vi "Display All Channels.vi"(0 "tagged llp packets cluster":T1, 1 "reset":bool, 2 "common resources":T11, 5 "serial channel display parameters":T23[](array[typedef])=[{"virtual channel"=0.0, "payload data type"=enum."Frame Start", "frame skip count"=0, "line skip count"=0, "pixel skip count"=0.0}, {"virtual channel"=0.0, "payload data type"=enum."Frame Start", "frame skip count"=0, "line skip count"=0, "pixel skip count"=0.0}, {"virtual channel"=0.0, "payload data type"=enum."Frame Start", "frame skip count"=0, "line skip count"=0, "pixel skip count"=0.0}, {"virtual channel"=0.0, "payload data type"=enum."Frame Start", "frame skip count"=0, "line skip count"=0, "pixel skip count"=0.0}, {"virtual channel"=0.0, "payload data type"=enum."Frame Start", "frame skip count"=0, "line skip count"=0, "pixel skip count"=0.0}, {"virtual channel"=0.0, "payload data type"=enum."Frame Start", "frame skip count"=0, "line skip count"=0, "pixel skip count"=0.0}, {"virtual channel"=0.0, "payload data type"=enum."Frame Start", "frame skip count"=0, "line skip count"=0, "pixel skip count"=0.0}, {"virtual channel"=0.0, "payload data type"=enum."Frame Start", "frame skip count"=0, "line skip count"=0, "pixel skip count"=0.0}], 7 "display serial channel selectors":fxp<+,3,3>[](array[numeric])=[0.0, 0.0, 0.0, 0.0, 0.0, 0.0, 0.0, 0.0], 9 "input valid":bool[](array[boolean])=[FALSE, FALSE, FALSE, FALSE, FALSE, FALSE, FALSE, FALSE], 11 "enabled display channels":bool[](array[boolean])=[FALSE, FALSE, FALSE, FALSE, FALSE, FALSE, FALSE, FALSE], 12 "gate display until frame complete":bool, 13 "num available display channels":fxp<+,4,4>=2.0) -> (4 "display channel status":T22[](array[typedef]), 14 "ready for input":bool[](array[boolean]))   [LabVIEW 2020, in "GettingStarted_Common_148X_FPGA.lvlib"]
uses:
  GettingStarted_Common_148X_FPGA.lvlib
  <instrlib>/FlexRIO/CSI-2/v2/FPGA/Types/Display Parameters.ctl
  <instrlib>/FlexRIO/CSI-2/v2/Common/Types/LLP Data Type.ctl
  Types/Display Channel Status.ctl
  Types/Common Resources.ctl
  <instrlib>/_niInstr/Memory/v1/FPGA/DRAM/niInstr Memory DRAM v1 FPGA.lvclass
  <instrlib>/FlexRIO/CSI-2/v2/FPGA/Types/Sync Pulse Resources.ctl
  Types/Serial Channel Resources.ctl
  Types/Single Serial Channel Resources.ctl
  <instrlib>/FlexRIO/CSI-2/v2/FPGA/DRAM Manager/Private/DRAM Manager.ctl
  <instrlib>/FlexRIO/CSI-2/v2/FPGA/DRAM Manager/Private/Common/DRAM Manager Registers.ctl
  <instrlib>/FlexRIO/CSI-2/v2/FPGA/DRAM Manager/Private/Common/Handshake Registers.ctl
  <instrlib>/FlexRIO/CSI-2/v2/FPGA/DRAM Manager/Private/Common/DRAM Manager FIFOs.ctl
  <instrlib>/FlexRIO/CSI-2/v2/FPGA/DRAM Manager/Private/Common/Write Data FIFO Ref.ctl
  <instrlib>/FlexRIO/CSI-2/v2/FPGA/DRAM Manager/Private/Common/Read Request Metadata FIFO Ref.ctl
  <instrlib>/FlexRIO/CSI-2/v2/FPGA/DRAM Manager/Private/Common/Read Data FIFO Ref.ctl
  Types/Tagged LLP Packets Cluster.ctl
  <instrlib>/FlexRIO/CSI-2/v2/FPGA/Types/Tagged LLP Packet.ctl
  <instrlib>/FlexRIO/CSI-2/v2/FPGA/Types/FPGA LLP Packet Tag.ctl
  <instrlib>/FlexRIO/CSI-2/v2/FPGA/Types/FPGA LLP Packet Timestamp.ctl
  <instrlib>/FlexRIO/CSI-2/v2/FPGA/Types/Timestamp ID.ctl
  <instrlib>/FlexRIO/CSI-2/v2/FPGA/Types/FPGA LLP Packet Size.ctl
  <instrlib>/FlexRIO/CSI-2/v2/FPGA/Types/LLP Packet.ctl
  <instrlib>/FlexRIO/CSI-2/v2/FPGA/Types/LLP Packet Header.ctl
  <instrlib>/FlexRIO/CSI-2/v2/FPGA/Types/LLP Packet Payload.ctl
  <instrlib>/FlexRIO/CSI-2/v2/FPGA/Types/LLP Packet Footer.ctl
  Types/Display Channel Resources.ctl
  <instrlib>/_niInstr/Basic Elements/v1/FPGA/niInstr Basic Elements v1 FPGA.lvlib
  <instrlib>/FlexRIO/CSI-2/v2/Common/NI CSI-2 API Common v2.lvlib
  <instrlib>/FlexRIO/CSI-2/v2/FPGA/NI CSI-2 API FPGA v2.lvlib
  <instrlib>/FlexRIO/CSI-2/v2/FPGA/DRAM Manager/DRAM Manager v2.lvlib
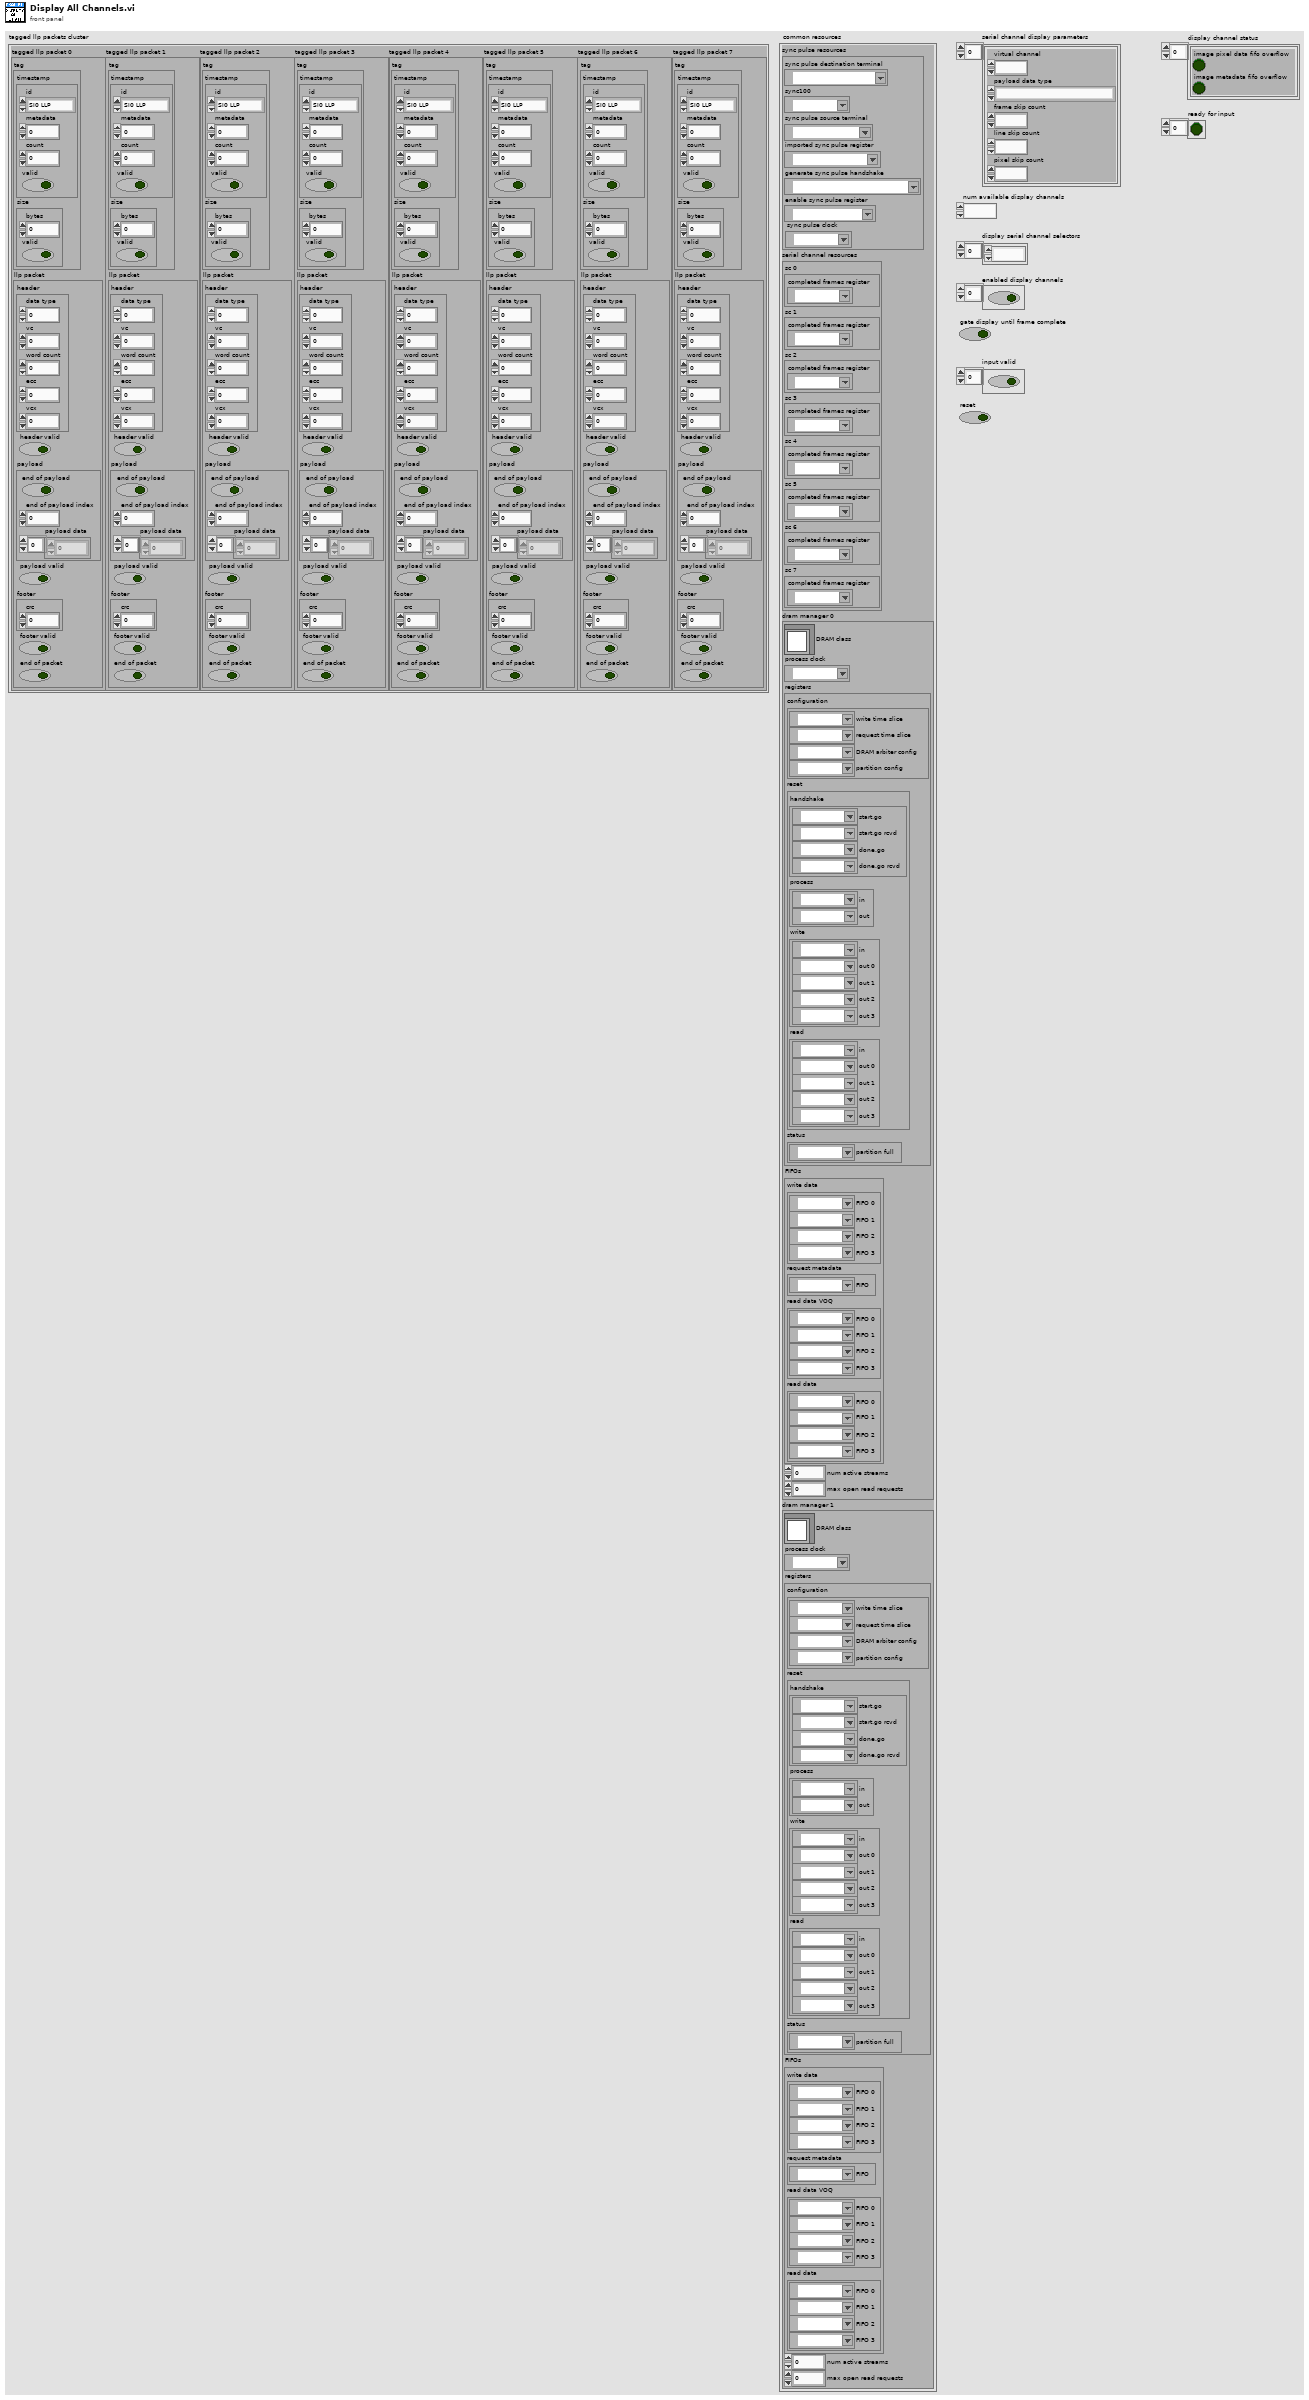
[diagram p1: front panel]
types:
  T1 = typedef "GettingStarted_Common_148X_FPGA.lvlib/Tagged LLP Packets Cluster.ctl" = cluster{"tagged llp packet 0":T2, "tagged llp packet 1":T2, "tagged llp packet 2":T2, "tagged llp packet 3":T2, "tagged llp packet 4":T2, "tagged llp packet 5":T2, "tagged llp packet 6":T2, "tagged llp packet 7":T2}
  T2 = typedef "NI CSI-2 API FPGA v2.lvlib/Tagged LLP Packet.ctl" = cluster{"tag":T3, "llp packet":T7}
  T3 = typedef "NI CSI-2 API FPGA v2.lvlib/FPGA LLP Packet Tag.ctl" = cluster{"timestamp":T4, "size":T6}
  T4 = typedef "NI CSI-2 API FPGA v2.lvlib/FPGA LLP Packet Timestamp.ctl" = cluster{"valid":bool, "count":fxp<+,50,50>, "id":T5, "metadata":u8}
  T5 = typedef "NI CSI-2 API FPGA v2.lvlib/Timestamp ID.ctl" = enum8{"SI0 LLP", "SI1 LLP", "SI2 LLP", "SI3 LLP", "SI4 LLP", "SI5 LLP", "SI6 LLP", "SI7 LLP", "SO0 LLP", "SO1 LLP", "SO2 LLP", "SO3 LLP", "SO4 LLP", "SO5 LLP", "SO6 LLP", "SO7 LLP", "Ser0 GPIO Bank", "Ser1 GPIO Bank", "Ser2 GPIO Bank", "Ser3 GPIO Bank", "Ser4 GPIO Bank", "Ser5 GPIO Bank", "Ser6 GPIO Bank", "Ser7 GPIO Bank", "Des0 GPIO Bank", "Des1 GPIO Bank", "Des2 GPIO Bank", "Des3 GPIO Bank", "Des4 GPIO Bank", "Des5 GPIO Bank", "Des6 GPIO Bank", "Des7 GPIO Bank", "User0", "User1", "User2", "User3", "User4", "User5", "User6", "User7", "User8", "User9", "User10", "User11", "User12", "User13", "User14", "User15", "User16", "User17", "User18", "User19", "User20", "User21", "User22", "User23", "User24", "User25", "User26", "User27", "User28", "User29", "User30", "User31"}
  T6 = typedef "NI CSI-2 API FPGA v2.lvlib/FPGA LLP Packet Size.ctl" = cluster{"bytes":fxp<+,17,17>, "valid":bool}
  T7 = typedef "NI CSI-2 API FPGA v2.lvlib/LLP Packet.ctl" = cluster{"header":T8, "header valid":bool, "payload":T9, "payload valid":bool, "footer":T10, "footer valid":bool, "end of packet":bool}
  T8 = typedef "NI CSI-2 API FPGA v2.lvlib/LLP Packet Header.ctl" = cluster{"word count":u16, "ecc":fxp<+,6,6>, "vcx":fxp<+,2,2>, "data type":fxp<+,6,6>, "vc":fxp<+,2,2>}
  T9 = typedef "NI CSI-2 API FPGA v2.lvlib/LLP Packet Payload.ctl" = cluster{"end of payload":bool, "end of payload index":fxp<+,3,3>, "payload data":u8[]}
  T10 = typedef "NI CSI-2 API FPGA v2.lvlib/LLP Packet Footer.ctl" = cluster{"crc":u16}
  T11 = typedef "GettingStarted_Common_148X_FPGA.lvlib/Common Resources.ctl" = cluster{"sync pulse resources":T12, "serial channel resources":T13, "dram manager 0":T15, "dram manager 1":T15}
  T12 = typedef "NI CSI-2 API FPGA v2.lvlib/Sync Pulse Resources.ctl" = cluster{"sync pulse destination terminal":refnum<k21>, "sync100":refnum<k21>, "sync pulse source terminal":refnum<k21>, "imported sync pulse register":refnum<k21>, "generate sync pulse handshake":refnum<k21>, "enable sync pulse register":refnum<k21>, "sync pulse clock":refnum<k21>}
  T13 = typedef "GettingStarted_Common_148X_FPGA.lvlib/Serial Channel Resources.ctl" = cluster{"sc 0":T14, "sc 1":T14, "sc 2":T14, "sc 3":T14, "sc 4":T14, "sc 5":T14, "sc 6":T14, "sc 7":T14}
  T14 = typedef "GettingStarted_Common_148X_FPGA.lvlib/Single Serial Channel Resources.ctl" = cluster{"completed frames register":refnum<k21>}
  T15 = typedef "DRAM Manager v2.lvlib/DRAM Manager.ctl" = cluster{"DRAM class":refnum<class "niInstr Memory DRAM v1 FPGA.lvclass">, "process clock":refnum<k21>, "registers":T16, "FIFOs":T18, "num active streams":fxp<+,3,3>, "max open read requests":u16}
  T16 = typedef "DRAM Manager v2.lvlib/DRAM Manager Registers.ctl" = cluster{"configuration":cluster{"write time slice":refnum<k21>, "request time slice":refnum<k21>, "DRAM arbiter config":refnum<k21>, "partition config":refnum<k21>}, "reset":cluster{"handshake":T17, "process":cluster{"in":refnum<k21>, "out":refnum<k21>}, "write":cluster{"in":refnum<k21>, "out 0":refnum<k21>, "out 1":refnum<k21>, "out 2":refnum<k21>, "out 3":refnum<k21>}, "read":cluster{"in":refnum<k21>, "out 0":refnum<k21>, "out 1":refnum<k21>, "out 2":refnum<k21>, "out 3":refnum<k21>}}, "status":cluster{"partition full":refnum<k21>}}
  T17 = typedef "DRAM Manager v2.lvlib/Handshake Registers.ctl" = cluster{"start.go":refnum<k21>, "start.go rcvd":refnum<k21>, "done.go":refnum<k21>, "done.go rcvd":refnum<k21>}
  T18 = typedef "DRAM Manager v2.lvlib/DRAM Manager FIFOs.ctl" = cluster{"write data":cluster{"FIFO 0":T19, "FIFO 1":T19, "FIFO 2":T19, "FIFO 3":T19}, "request metadata":cluster{"FIFO":T20}, "read data VOQ":cluster{"FIFO 0":T21, "FIFO 1":T21, "FIFO 2":T21, "FIFO 3":T21}, "read data":cluster{"FIFO 0":T21, "FIFO 1":T21, "FIFO 2":T21, "FIFO 3":T21}}
  T19 = typedef "DRAM Manager v2.lvlib/Write Data FIFO Ref.ctl" = refnum<k21>
  T20 = typedef "DRAM Manager v2.lvlib/Read Request Metadata FIFO Ref.ctl" = refnum<k21>
  T21 = typedef "DRAM Manager v2.lvlib/Read Data FIFO Ref.ctl" = refnum<k21>
  T22 = typedef "GettingStarted_Common_148X_FPGA.lvlib/Display Channel Status.ctl" = cluster{"image pixel data fifo overflow":bool, "image metadata fifo overflow":bool}
  T23 = typedef "NI CSI-2 API FPGA v2.lvlib/Display Parameters.ctl" = cluster{"virtual channel":fxp<+,4,4>, "payload data type":T24, "frame skip count":u16, "line skip count":u8, "pixel skip count":fxp<+,5,5>}
  T24 = typedef "NI CSI-2 API Common v2.lvlib/LLP Data Type.ctl" = enum8{"Frame Start", "Frame End", "Line Start", "Line End", "End of Transmission", "Reserved 0", "Reserved 1", "Reserved 2", "Generic Short Packet 1", "Generic Short Packet 2", "Generic Short Packet 3", "Generic Short Packet 4", "Generic Short Packet 5", "Generic Short Packet 6", "Generic Short Packet 7", "Generic Short Packet 8", "Null", "Blanking Data", "Embedded 8-bit non Image Data", "Generic Long Packet 1", "Generic Long Packet 2", "Generic Long Packet 3", "Generic Long Packet 4", "Reserved 3", "YUV420 8-bit", "YUV420 10-bit", "Legacy YUV420 8-bit", "Reserved 4", "YUV420 8-bit Chroma Shifted", "YUV420 10-bit Chroma Shifted", "YUV422 8-bit", "YUV422 10-bit", "RGB444", "RGB555", "RGB565", "RGB666", "RGB888", "Reserved 5", "Reserved 6", "RAW 24", "RAW 6", "RAW 7", "RAW 8", "RAW 10", "RAW 12", "RAW 14", "RAW 16", "RAW 20", "User Defined 8-bit Data 1", "User Defined 8-bit Data 2", "User Defined 8-bit Data 3", "User Defined 8-bit Data 4", "User Defined 8-bit Data 5", "User Defined 8-bit Data 6", "User Defined 8-bit Data 7", "User Defined 8-bit Data 8", "USL Command", "Reserved 7", "Reserved 8", "Reserved 9", "Reserved 10", "Reserved 11", "Reserved 12", "LRTE EPD Spacer"}
  T25 = typedef "GettingStarted_Common_148X_FPGA.lvlib/Display Channel Resources.ctl" = cluster{"image pixel data dma fifo x8":refnum<k21>, "image pixel data dma fifo x16":refnum<k21>, "image metadata dma fifo":refnum<k21>, "serial channel resources":T13}
  T26 = cluster{"gate display until frame complete":bool, "reset":bool, "serial channel display parameters":T23[], "tagged llp packets cluster":T1, "output valid":bool[], "display channel resources":cluster{"display resources 0":T25, "display resources 1":T25, "display resources 2":T25, "display resources 3":T25, "display resources 4":T25, "display resources 5":T25, "display resources 6":T25, "display resources 7":T25}}
  T27 = cluster{"channel selector":fxp<+,3,3>, "enabled display channels":bool}
  T28 = cluster{"display resources 0":T25, "display resources 1":T25, "display resources 2":T25, "display resources 3":T25, "display resources 4":T25, "display resources 5":T25, "display resources 6":T25, "display resources 7":T25}
  T29 = cluster{"display channel status":T22, "selected channel":fxp<+,3,3>, "ready for input":bool, "enabled display channels":bool}
  T30 = cluster{"display channel status":T22, "selected channel":fxp<+,3,3>, "ready for input":bool, "enabled display channels":bool}[]
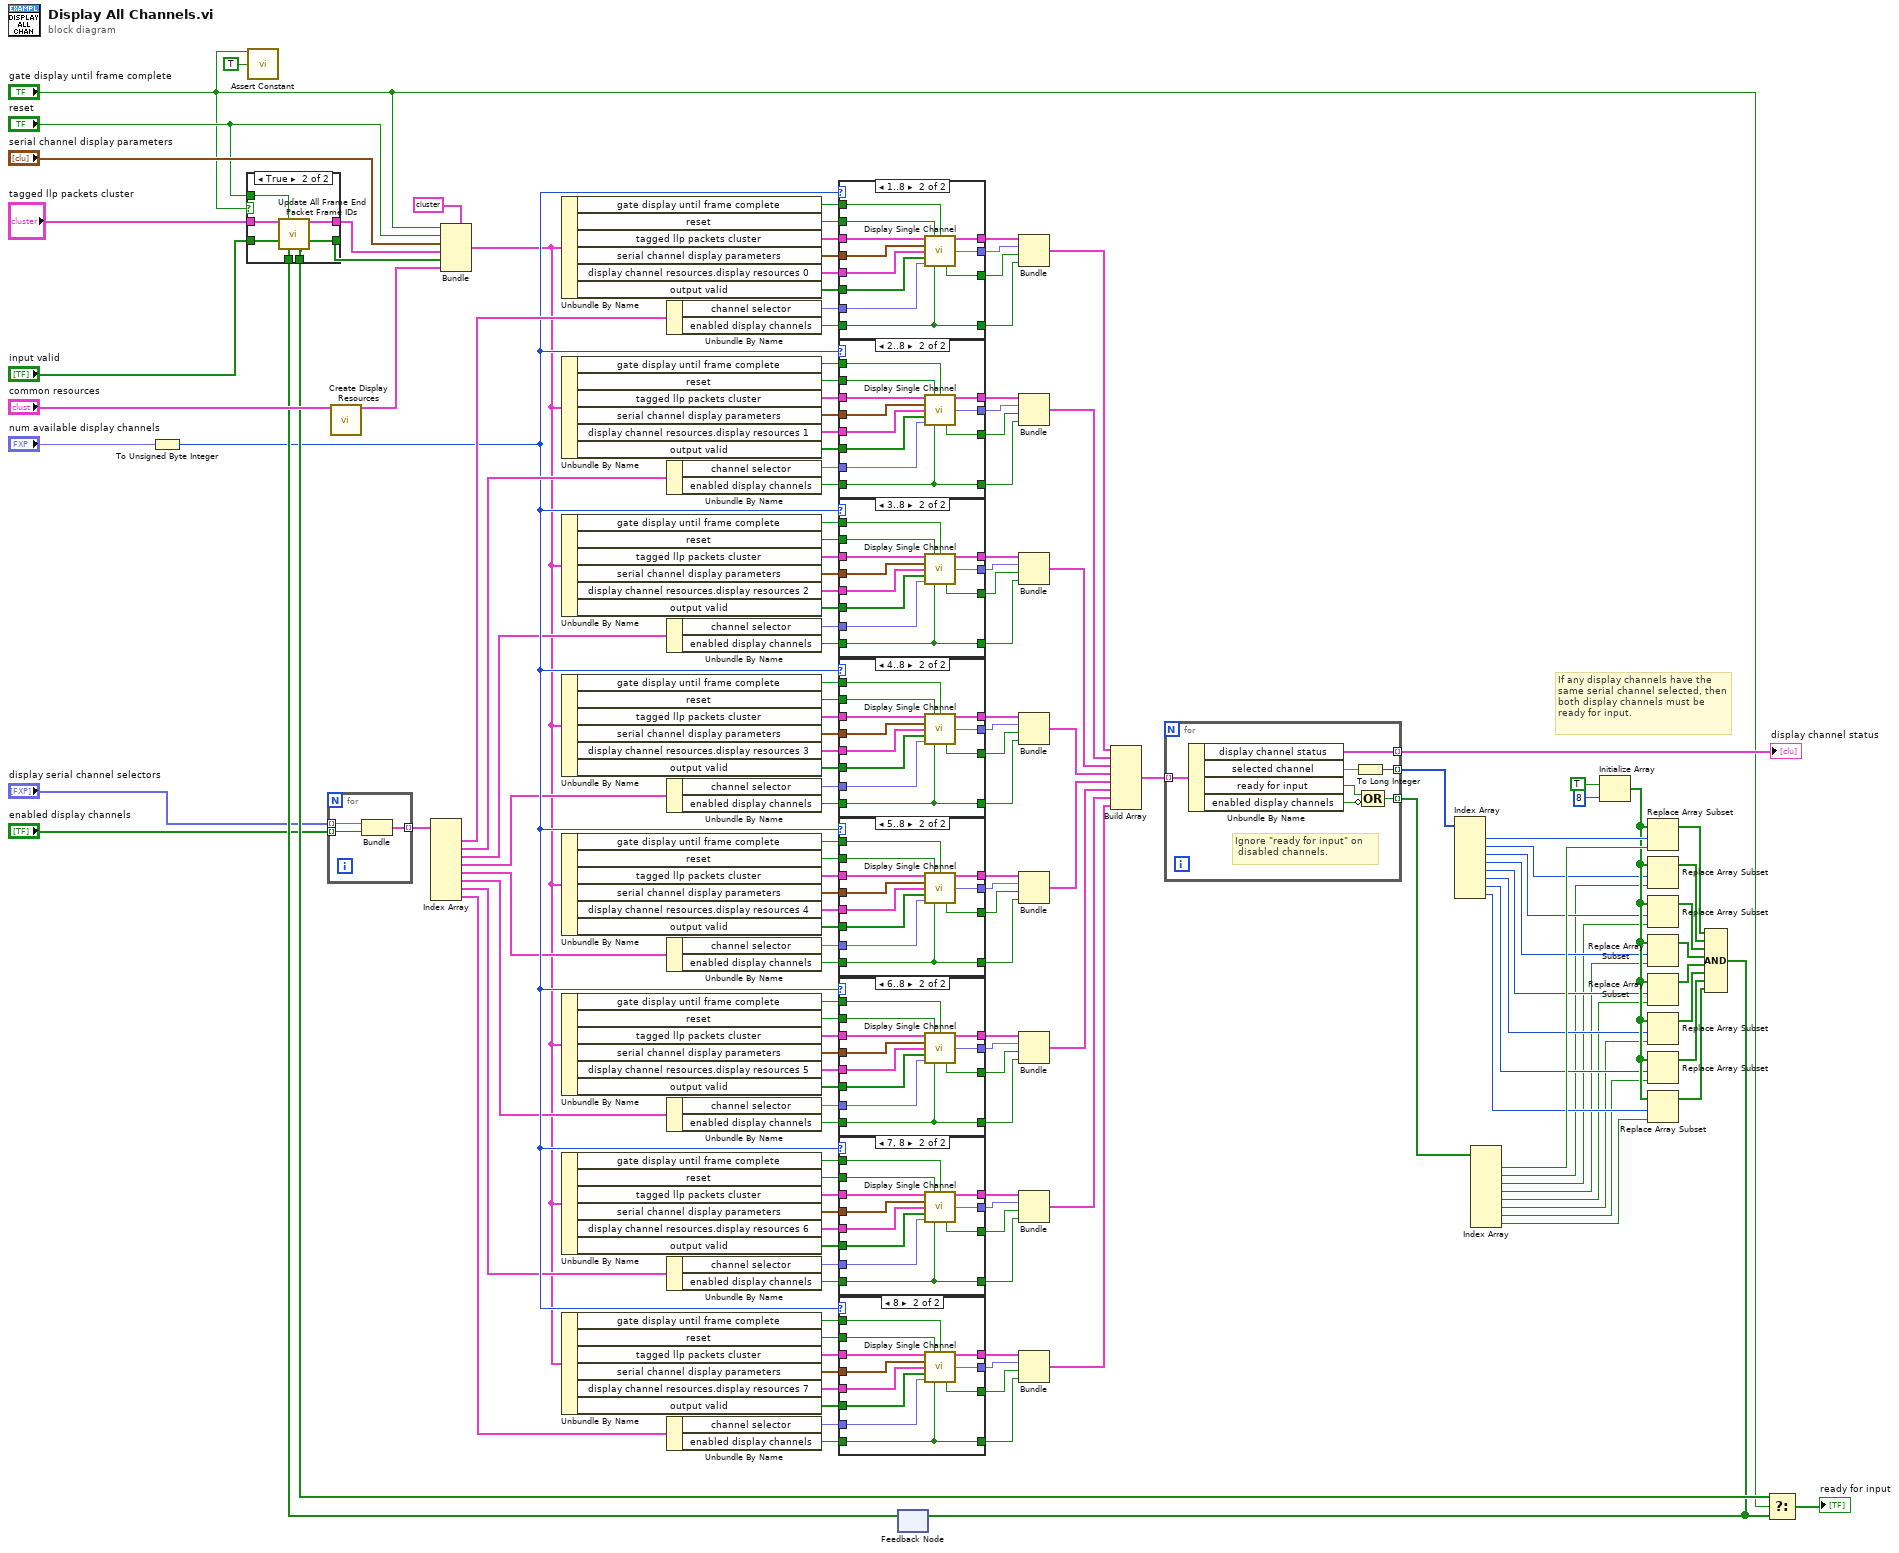
[diagram p0: block diagram]
diagram:
  # "If any display channels have the same serial channel selected, then both display channels must be ready for input."
  n1 = To Unsigned Byte Integer(number="num available display channels") -> (unsigned 8bit integer=w85:u8)
  n2 = call <instrlib>:"Assert Constant.vi"("constant terminal"="gate display until frame complete", "enable show error"=TRUE) -> ()  [unwired: 14 in]
  n3 = for {
    tunnel: "enabled display channels" -> [w166] mode=indexing
    tunnel: "display serial channel selectors" -> [w167] mode=indexing
    tunnel: [w165] -> w105 mode=indexing
    n4 = Bundle("channel selector"=w167, "enabled display channels"=w166) -> (w165:T27)  [unwired: 1 in]
  }
  n5 = call "Create Display Resources.vi"("common resources"="common resources") -> ("display channel resources"=w112:T28)  [unwired: 14 in]
  n6 = Index Array(array=w105) -> (element #1=w104:T27, element #2=w86:T27, element #3=w18:T27, element #4=w17:T27, element #5=w16:T27, element #6=w13:T27, element #7=w15:T27, element #8=w14:T27)  [unwired: 8 in]
  n7 = Unbundle By Name(w104) -> ("channel selector"=w102:fxp<+,3,3>, "enabled display channels"=w103:bool)
  n8 = Unbundle By Name(w86) -> ("channel selector"=w91:fxp<+,3,3>, "enabled display channels"=w90:bool)
  n9 = Unbundle By Name(w18) -> ("channel selector"=w73:fxp<+,3,3>, "enabled display channels"=w72:bool)
  n10 = Unbundle By Name(w17) -> ("channel selector"=w66:fxp<+,3,3>, "enabled display channels"=w65:bool)
  n11 = Unbundle By Name(w16) -> ("channel selector"=w50:fxp<+,3,3>, "enabled display channels"=w49:bool)
  n12 = Unbundle By Name(w13) -> ("channel selector"=w43:fxp<+,3,3>, "enabled display channels"=w42:bool)
  n13 = Unbundle By Name(w15) -> ("channel selector"=w27:fxp<+,3,3>, "enabled display channels"=w26:bool)
  n14 = Unbundle By Name(w14) -> ("channel selector"=w20:fxp<+,3,3>, "enabled display channels"=w19:bool)
  n15 = feedback #1() -> (w159:bool[])  [unwired: 1 in]
  n16 = case shown="True" "gate display until frame complete" {
    tunnel: "reset" -> [_ w176]
    tunnel: "input valid" -> [w168 w175]
    tunnel: [w168 w174] -> w113
    tunnel: "tagged llp packets cluster" -> [w169 w173]
    tunnel: [w169 w172] -> w110
    tunnel: [_ w171] -> w158
    tunnel: w159 -> [_ w170]
    frame False {
    }
    frame True {
      n17 = call "Update All Frame End Packet Frame IDs.vi"("tagged llp packets cluster"=w173, "reset"=w176, "input valid"=w175, "ready for output"=w170) -> ("tagged llp packets cluster"=w172:T1, "output valid"=w174:bool[], "ready for input"=w171:bool[])  [unwired: 9 in]
    }
  }
  n18 = Bundle(cluster=T26 {"gate display until frame complete"=FALSE, "reset"=FALSE, "serial channel display parameters"=[{"virtual channel"=0.0, "payload data type"=enum."Frame Start", "frame skip count"=0, "line skip count"=0, "pixel skip count"=0.0}, {"virtual channel"=0.0, "payload data type"=enum."Frame Start", "frame skip count"=0, "line skip count"=0, "pixel skip count"=0.0}, {"virtual channel"=0.0, "payload data type"=enum."Frame Start", "frame skip count"=0, "line skip count"=0, "pixel skip count"=0.0}, {"virtual channel"=0.0, "payload data type"=enum."Frame Start", "frame skip count"=0, "line skip count"=0, "pixel skip count"=0.0}, {"virtual channel"=0.0, "payload data type"=enum."Frame Start", "frame skip count"=0, "line skip count"=0, "pixel skip count"=0.0}, {"virtual channel"=0.0, "payload data type"=enum."Frame Start", "frame skip count"=0, "line skip count"=0, "pixel skip count"=0.0}, {"virtual channel"=0.0, "payload data type"=enum."Frame Start", "frame skip count"=0, "line skip count"=0, "pixel skip count"=0.0}, {"virtual channel"=0.0, "payload data type"=enum."Frame Start", "frame skip count"=0, "line skip count"=0, "pixel skip count"=0.0}], "tagged llp packets cluster"={"tagged llp packet 0"={"tag"={"timestamp"={"valid"=FALSE, "count"=0.0, "id"=enum."SI0 LLP", "metadata"=0}, "size"={"bytes"=0.0, "valid"=FALSE}}, "llp packet"={"header"={"word count"=0, "ecc"=0.0, "vcx"=0.0, "data type"=0.0, "vc"=0.0}, "header valid"=FALSE, "payload"={"end of payload"=FALSE, "end of payload index"=0.0, "payload data"=[]}, "payload valid"=FALSE, "footer"={"crc"=0}, "footer valid"=FALSE, "end of packet"=FALSE}}, "tagged llp packet 1"={"tag"={"timestamp"={"valid"=FALSE, "count"=0.0, "id"=enum."SI0 LLP", "metadata"=0}, "size"={"bytes"=0.0, "valid"=FALSE}}, "llp packet"={"header"={"word count"=0, "ecc"=0.0, "vcx"=0.0, "data type"=0.0, "vc"=0.0}, "header valid"=FALSE, "payload"={"end of payload"=FALSE, "end of payload index"=0.0, "payload data"=[]}, "payload valid"=FALSE, "footer"={"crc"=0}, "footer valid"=FALSE, "end of packet"=FALSE}}, "tagged llp packet 2"={"tag"={"timestamp"={"valid"=FALSE, "count"=0.0, "id"=enum."SI0 LLP", "metadata"=0}, "size"={"bytes"=0.0, "valid"=FALSE}}, "llp packet"={"header"={"word count"=0, "ecc"=0.0, "vcx"=0.0, "data type"=0.0, "vc"=0.0}, "header valid"=FALSE, "payload"={"end of payload"=FALSE, "end of payload index"=0.0, "payload data"=[]}, "payload valid"=FALSE, "footer"={"crc"=0}, "footer valid"=FALSE, "end of packet"=FALSE}}, "tagged llp packet 3"={"tag"={"timestamp"={"valid"=FALSE, "count"=0.0, "id"=enum."SI0 LLP", "metadata"=0}, "size"={"bytes"=0.0, "valid"=FALSE}}, "llp packet"={"header"={"word count"=0, "ecc"=0.0, "vcx"=0.0, "data type"=0.0, "vc"=0.0}, "header valid"=FALSE, "payload"={"end of payload"=FALSE, "end of payload index"=0.0, "payload data"=[]}, "payload valid"=FALSE, "footer"={"crc"=0}, "footer valid"=FALSE, "end of packet"=FALSE}}, "tagged llp packet 4"={"tag"={"timestamp"={"valid"=FALSE, "count"=0.0, "id"=enum."SI0 LLP", "metadata"=0}, "size"={"bytes"=0.0, "valid"=FALSE}}, "llp packet"={"header"={"word count"=0, "ecc"=0.0, "vcx"=0.0, "data type"=0.0, "vc"=0.0}, "header valid"=FALSE, "payload"={"end of payload"=FALSE, "end of payload index"=0.0, "payload data"=[]}, "payload valid"=FALSE, "footer"={"crc"=0}, "footer valid"=FALSE, "end of packet"=FALSE}}, "tagged llp packet 5"={"tag"={"timestamp"={"valid"=FALSE, "count"=0.0, "id"=enum."SI0 LLP", "metadata"=0}, "size"={"bytes"=0.0, "valid"=FALSE}}, "llp packet"={"header"={"word count"=0, "ecc"=0.0, "vcx"=0.0, "data type"=0.0, "vc"=0.0}, "header valid"=FALSE, "payload"={"end of payload"=FALSE, "end of payload index"=0.0, "payload data"=[]}, "payload valid"=FALSE, "footer"={"crc"=0}, "footer valid"=FALSE, "end of packet"=FALSE}}, "tagged llp packet 6"={"tag"={"timestamp"={"valid"=FALSE, "count"=0.0, "id"=enum."SI0 LLP", "metadata"=0}, "size"={"bytes"=0.0, "valid"=FALSE}}, "llp packet"={"header"={"word count"=0, "ecc"=0.0, "vcx"=0.0, "data type"=0.0, "vc"=0.0}, "header valid"=FALSE, "payload"={"end of payload"=FALSE, "end of payload index"=0.0, "payload data"=[]}, "payload valid"=FALSE, "footer"={"crc"=0}, "footer valid"=FALSE, "end of packet"=FALSE}}, "tagged llp packet 7"={"tag"={"timestamp"={"valid"=FALSE, "count"=0.0, "id"=enum."SI0 LLP", "metadata"=0}, "size"={"bytes"=0.0, "valid"=FALSE}}, "llp packet"={"header"={"word count"=0, "ecc"=0.0, "vcx"=0.0, "data type"=0.0, "vc"=0.0}, "header valid"=FALSE, "payload"={"end of payload"=FALSE, "end of payload index"=0.0, "payload data"=[]}, "payload valid"=FALSE, "footer"={"crc"=0}, "footer valid"=FALSE, "end of packet"=FALSE}}}, "output valid"=[FALSE, FALSE, FALSE, FALSE, FALSE, FALSE, FALSE, FALSE], "display channel resources"={"display resources 0"={"image pixel data dma fifo x8"="", "image pixel data dma fifo x16"="", "image metadata dma fifo"="", "serial channel resources"={"sc 0"={"completed frames register"=""}, "sc 1"={"completed frames register"=""}, "sc 2"={"completed frames register"=""}, "sc 3"={"completed frames register"=""}, "sc 4"={"completed frames register"=""}, "sc 5"={"completed frames register"=""}, "sc 6"={"completed frames register"=""}, "sc 7"={"completed frames register"=""}}}, "display resources 1"={"image pixel data dma fifo x8"="", "image pixel data dma fifo x16"="", "image metadata dma fifo"="", "serial channel resources"={"sc 0"={"completed frames register"=""}, "sc 1"={"completed frames register"=""}, "sc 2"={"completed frames register"=""}, "sc 3"={"completed frames register"=""}, "sc 4"={"completed frames register"=""}, "sc 5"={"completed frames register"=""}, "sc 6"={"completed frames register"=""}, "sc 7"={"completed frames register"=""}}}, "display resources 2"={"image pixel data dma fifo x8"="", "image pixel data dma fifo x16"="", "image metadata dma fifo"="", "serial channel resources"={"sc 0"={"completed frames register"=""}, "sc 1"={"completed frames register"=""}, "sc 2"={"completed frames register"=""}, "sc 3"={"completed frames register"=""}, "sc 4"={"completed frames register"=""}, "sc 5"={"completed frames register"=""}, "sc 6"={"completed frames register"=""}, "sc 7"={"completed frames register"=""}}}, "display resources 3"={"image pixel data dma fifo x8"="", "image pixel data dma fifo x16"="", "image metadata dma fifo"="", "serial channel resources"={"sc 0"={"completed frames register"=""}, "sc 1"={"completed frames register"=""}, "sc 2"={"completed frames register"=""}, "sc 3"={"completed frames register"=""}, "sc 4"={"completed frames register"=""}, "sc 5"={"completed frames register"=""}, "sc 6"={"completed frames register"=""}, "sc 7"={"completed frames register"=""}}}, "display resources 4"={"image pixel data dma fifo x8"="", "image pixel data dma fifo x16"="", "image metadata dma fifo"="", "serial channel resources"={"sc 0"={"completed frames register"=""}, "sc 1"={"completed frames register"=""}, "sc 2"={"completed frames register"=""}, "sc 3"={"completed frames register"=""}, "sc 4"={"completed frames register"=""}, "sc 5"={"completed frames register"=""}, "sc 6"={"completed frames register"=""}, "sc 7"={"completed frames register"=""}}}, "display resources 5"={"image pixel data dma fifo x8"="", "image pixel data dma fifo x16"="", "image metadata dma fifo"="", "serial channel resources"={"sc 0"={"completed frames register"=""}, "sc 1"={"completed frames register"=""}, "sc 2"={"completed frames register"=""}, "sc 3"={"completed frames register"=""}, "sc 4"={"completed frames register"=""}, "sc 5"={"completed frames register"=""}, "sc 6"={"completed frames register"=""}, "sc 7"={"completed frames register"=""}}}, "display resources 6"={"image pixel data dma fifo x8"="", "image pixel data dma fifo x16"="", "image metadata dma fifo"="", "serial channel resources"={"sc 0"={"completed frames register"=""}, "sc 1"={"completed frames register"=""}, "sc 2"={"completed frames register"=""}, "sc 3"={"completed frames register"=""}, "sc 4"={"completed frames register"=""}, "sc 5"={"completed frames register"=""}, "sc 6"={"completed frames register"=""}, "sc 7"={"completed frames register"=""}}}, "display resources 7"={"image pixel data dma fifo x8"="", "image pixel data dma fifo x16"="", "image metadata dma fifo"="", "serial channel resources"={"sc 0"={"completed frames register"=""}, "sc 1"={"completed frames register"=""}, "sc 2"={"completed frames register"=""}, "sc 3"={"completed frames register"=""}, "sc 4"={"completed frames register"=""}, "sc 5"={"completed frames register"=""}, "sc 6"={"completed frames register"=""}, "sc 7"={"completed frames register"=""}}}}} ("output cluster"), "gate display until frame complete"="gate display until frame complete", "reset"="reset", "serial channel display parameters"="serial channel display parameters", "tagged llp packets cluster"=w110, "output valid"=w113, "display channel resources"=w112) -> (w12:T26)
  n19 = Unbundle By Name(w12) -> ("gate display until frame complete"=w99:bool, "reset"=w98:bool, "tagged llp packets cluster"=w109:T1, "serial channel display parameters"=w108:T23[], "display channel resources.display resources 0"=w107:T25, "output valid"=w106:bool[])
  n20 = Unbundle By Name(w12) -> ("gate display until frame complete"=w97:bool, "reset"=w96:bool, "tagged llp packets cluster"=w95:T1, "serial channel display parameters"=w94:T23[], "display channel resources.display resources 1"=w93:T25, "output valid"=w92:bool[])
  n21 = Unbundle By Name(w12) -> ("gate display until frame complete"=w84:bool, "reset"=w78:bool, "tagged llp packets cluster"=w77:T1, "serial channel display parameters"=w76:T23[], "display channel resources.display resources 2"=w75:T25, "output valid"=w74:bool[])
  n22 = Unbundle By Name(w12) -> ("gate display until frame complete"=w83:bool, "reset"=w71:bool, "tagged llp packets cluster"=w70:T1, "serial channel display parameters"=w69:T23[], "display channel resources.display resources 3"=w68:T25, "output valid"=w67:bool[])
  n23 = Unbundle By Name(w12) -> ("gate display until frame complete"=w82:bool, "reset"=w55:bool, "tagged llp packets cluster"=w54:T1, "serial channel display parameters"=w53:T23[], "display channel resources.display resources 4"=w52:T25, "output valid"=w51:bool[])
  n24 = Unbundle By Name(w12) -> ("gate display until frame complete"=w81:bool, "reset"=w48:bool, "tagged llp packets cluster"=w47:T1, "serial channel display parameters"=w46:T23[], "display channel resources.display resources 5"=w45:T25, "output valid"=w44:bool[])
  n25 = Unbundle By Name(w12) -> ("gate display until frame complete"=w79:bool, "reset"=w32:bool, "tagged llp packets cluster"=w31:T1, "serial channel display parameters"=w30:T23[], "display channel resources.display resources 6"=w29:T25, "output valid"=w28:bool[])
  n26 = Unbundle By Name(w12) -> ("gate display until frame complete"=w80:bool, "reset"=w25:bool, "tagged llp packets cluster"=w24:T1, "serial channel display parameters"=w23:T23[], "display channel resources.display resources 7"=w22:T25, "output valid"=w21:bool[])
  n27 = case shown="1..8" w85 {
    tunnel: w103 -> [_ w177]
    tunnel: [_ w185] -> w155
    tunnel: w98 -> [_ w184]
    tunnel: w99 -> [_ w183]
    tunnel: [_ w187] -> w153
    tunnel: w102 -> [_ w180]
    tunnel: [_ w186] -> w154
    tunnel: w109 -> [_ w182]
    tunnel: w108 -> [_ w181]
    tunnel: w107 -> [_ w178]
    tunnel: w106 -> [_ w179]
    tunnel: [_ w177] -> w9
    frame Default {
    }
    frame 1..8 {
      n28 = call "Display Single Channel.vi"("tagged llp packets cluster"=w182, "reset"=w184, "gate display until frame complete"=w183, "display parameters in"=w181, "display resources"=w178, "input valid"=w179, "channel selector"=w180, "enable channel"=w177) -> ("display channel status"=w185:T22, "selected channel"=w186:fxp<+,3,3>, "ready for input"=w187:bool)  [unwired: 5 in]
    }
  }
  n29 = case shown="2..8" w85 {
    tunnel: w90 -> [_ w188]
    tunnel: [_ w196] -> w89
    tunnel: w96 -> [_ w195]
    tunnel: w97 -> [_ w194]
    tunnel: [_ w198] -> w87
    tunnel: w91 -> [_ w191]
    tunnel: [_ w197] -> w88
    tunnel: w95 -> [_ w193]
    tunnel: w94 -> [_ w192]
    tunnel: w93 -> [_ w189]
    tunnel: w92 -> [_ w190]
    tunnel: [_ w188] -> w8
    frame Default {
    }
    frame 2..8 {
      n30 = call "Display Single Channel.vi"("tagged llp packets cluster"=w193, "reset"=w195, "gate display until frame complete"=w194, "display parameters in"=w192, "display resources"=w189, "input valid"=w190, "channel selector"=w191, "enable channel"=w188) -> ("display channel status"=w196:T22, "selected channel"=w197:fxp<+,3,3>, "ready for input"=w198:bool)  [unwired: 5 in]
    }
  }
  n31 = case shown="3..8" w85 {
    tunnel: w72 -> [_ w199]
    tunnel: [_ w207] -> w64
    tunnel: w78 -> [_ w206]
    tunnel: w84 -> [_ w205]
    tunnel: [_ w209] -> w62
    tunnel: w73 -> [_ w202]
    tunnel: [_ w208] -> w63
    tunnel: w77 -> [_ w204]
    tunnel: w76 -> [_ w203]
    tunnel: w75 -> [_ w200]
    tunnel: w74 -> [_ w201]
    tunnel: [_ w199] -> w11
    frame Default {
    }
    frame 3..8 {
      n32 = call "Display Single Channel.vi"("tagged llp packets cluster"=w204, "reset"=w206, "gate display until frame complete"=w205, "display parameters in"=w203, "display resources"=w200, "input valid"=w201, "channel selector"=w202, "enable channel"=w199) -> ("display channel status"=w207:T22, "selected channel"=w208:fxp<+,3,3>, "ready for input"=w209:bool)  [unwired: 5 in]
    }
  }
  n33 = case shown="4..8" w85 {
    tunnel: w65 -> [_ w210]
    tunnel: [_ w218] -> w61
    tunnel: w71 -> [_ w217]
    tunnel: w83 -> [_ w216]
    tunnel: [_ w220] -> w59
    tunnel: w66 -> [_ w213]
    tunnel: [_ w219] -> w60
    tunnel: w70 -> [_ w215]
    tunnel: w69 -> [_ w214]
    tunnel: w68 -> [_ w211]
    tunnel: w67 -> [_ w212]
    tunnel: [_ w210] -> w7
    frame Default {
    }
    frame 4..8 {
      n34 = call "Display Single Channel.vi"("tagged llp packets cluster"=w215, "reset"=w217, "gate display until frame complete"=w216, "display parameters in"=w214, "display resources"=w211, "input valid"=w212, "channel selector"=w213, "enable channel"=w210) -> ("display channel status"=w218:T22, "selected channel"=w219:fxp<+,3,3>, "ready for input"=w220:bool)  [unwired: 5 in]
    }
  }
  n35 = case shown="5..8" w85 {
    tunnel: w49 -> [_ w221]
    tunnel: [_ w229] -> w58
    tunnel: w55 -> [_ w228]
    tunnel: w82 -> [_ w227]
    tunnel: [_ w231] -> w56
    tunnel: w50 -> [_ w224]
    tunnel: [_ w230] -> w57
    tunnel: w54 -> [_ w226]
    tunnel: w53 -> [_ w225]
    tunnel: w52 -> [_ w222]
    tunnel: w51 -> [_ w223]
    tunnel: [_ w221] -> w6
    frame Default {
    }
    frame 5..8 {
      n36 = call "Display Single Channel.vi"("tagged llp packets cluster"=w226, "reset"=w228, "gate display until frame complete"=w227, "display parameters in"=w225, "display resources"=w222, "input valid"=w223, "channel selector"=w224, "enable channel"=w221) -> ("display channel status"=w229:T22, "selected channel"=w230:fxp<+,3,3>, "ready for input"=w231:bool)  [unwired: 5 in]
    }
  }
  n37 = case shown="6..8" w85 {
    tunnel: w42 -> [_ w232]
    tunnel: [_ w240] -> w41
    tunnel: w48 -> [_ w239]
    tunnel: w81 -> [_ w238]
    tunnel: [_ w242] -> w33
    tunnel: w43 -> [_ w235]
    tunnel: [_ w241] -> w34
    tunnel: w47 -> [_ w237]
    tunnel: w46 -> [_ w236]
    tunnel: w45 -> [_ w233]
    tunnel: w44 -> [_ w234]
    tunnel: [_ w232] -> w5
    frame Default {
    }
    frame 6..8 {
      n38 = call "Display Single Channel.vi"("tagged llp packets cluster"=w237, "reset"=w239, "gate display until frame complete"=w238, "display parameters in"=w236, "display resources"=w233, "input valid"=w234, "channel selector"=w235, "enable channel"=w232) -> ("display channel status"=w240:T22, "selected channel"=w241:fxp<+,3,3>, "ready for input"=w242:bool)  [unwired: 5 in]
    }
  }
  n39 = case shown="7, 8" w85 {
    tunnel: w26 -> [_ w243]
    tunnel: [_ w251] -> w40
    tunnel: w32 -> [_ w250]
    tunnel: w79 -> [_ w249]
    tunnel: [_ w253] -> w35
    tunnel: w27 -> [_ w246]
    tunnel: [_ w252] -> w36
    tunnel: w31 -> [_ w248]
    tunnel: w30 -> [_ w247]
    tunnel: w29 -> [_ w244]
    tunnel: w28 -> [_ w245]
    tunnel: [_ w243] -> w4
    frame Default {
    }
    frame 7, 8 {
      n40 = call "Display Single Channel.vi"("tagged llp packets cluster"=w248, "reset"=w250, "gate display until frame complete"=w249, "display parameters in"=w247, "display resources"=w244, "input valid"=w245, "channel selector"=w246, "enable channel"=w243) -> ("display channel status"=w251:T22, "selected channel"=w252:fxp<+,3,3>, "ready for input"=w253:bool)  [unwired: 5 in]
    }
  }
  n41 = case shown="8" w85 {
    tunnel: w19 -> [_ w254]
    tunnel: [_ w262] -> w39
    tunnel: w25 -> [_ w261]
    tunnel: w80 -> [_ w260]
    tunnel: [_ w264] -> w37
    tunnel: w20 -> [_ w257]
    tunnel: [_ w263] -> w38
    tunnel: w24 -> [_ w259]
    tunnel: w23 -> [_ w258]
    tunnel: w22 -> [_ w255]
    tunnel: w21 -> [_ w256]
    tunnel: [_ w254] -> w3
    frame Default {
    }
    frame 8 {
      n42 = call "Display Single Channel.vi"("tagged llp packets cluster"=w259, "reset"=w261, "gate display until frame complete"=w260, "display parameters in"=w258, "display resources"=w255, "input valid"=w256, "channel selector"=w257, "enable channel"=w254) -> ("display channel status"=w262:T22, "selected channel"=w263:fxp<+,3,3>, "ready for input"=w264:bool)  [unwired: 5 in]
    }
  }
  n43 = Bundle("display channel status"=w155, "selected channel"=w154, "ready for input"=w153, "enabled display channels"=w9) -> (w152:T29)  [unwired: 1 in]
  n44 = Bundle("display channel status"=w89, "selected channel"=w88, "ready for input"=w87, "enabled display channels"=w8) -> (w149:T29)  [unwired: 1 in]
  n45 = Bundle("display channel status"=w64, "selected channel"=w63, "ready for input"=w62, "enabled display channels"=w11) -> (w148:T29)  [unwired: 1 in]
  n46 = Bundle("display channel status"=w61, "selected channel"=w60, "ready for input"=w59, "enabled display channels"=w7) -> (w147:T29)  [unwired: 1 in]
  n47 = Bundle("display channel status"=w58, "selected channel"=w57, "ready for input"=w56, "enabled display channels"=w6) -> (w146:T29)  [unwired: 1 in]
  n48 = Bundle("display channel status"=w41, "selected channel"=w34, "ready for input"=w33, "enabled display channels"=w5) -> (w145:T29)  [unwired: 1 in]
  n49 = Bundle("display channel status"=w40, "selected channel"=w36, "ready for input"=w35, "enabled display channels"=w4) -> (w143:T29)  [unwired: 1 in]
  n50 = Bundle("display channel status"=w39, "selected channel"=w38, "ready for input"=w37, "enabled display channels"=w3) -> (w144:T29)  [unwired: 1 in]
  n51 = Build Array(w152, w149, w148, w147, w146, w145, w143, w144) -> (w151:T30)
  n52 = for {
    tunnel: w151 -> [w271] mode=indexing
    tunnel: [w270] -> w150 mode=indexing
    tunnel: [w268] -> w142 mode=indexing
    tunnel: [w265] -> w10 mode=indexing
    # "Ignore \"ready for input\" on\n disabled channels."
    n53 = Unbundle By Name(w271) -> ("display channel status"=w270:T22, "selected channel"=w269:fxp<+,3,3>, "ready for input"=w267:bool, "enabled display channels"=w266:bool)
    n54 = To Long Integer(number=w269) -> (32bit integer=w268:i32)
    n55 = Compound Arithmetic op=OR(w267, invert w266) -> (w265:bool)
  }
  "display channel status" <- w150
  n56 = Index Array(array=w142) -> (element #1=w141:i32, element #2=w130:i32, element #3=w129:i32, element #4=w128:i32, element #5=w127:i32, element #6=w126:i32, element #7=w125:i32, element #8=w124:i32)  [unwired: 8 in]
  n57 = Index Array(array=w10) -> (element #1=w140:bool, element #2=w123:bool, element #3=w117:bool, element #4=w118:bool, element #5=w119:bool, element #6=w120:bool, element #7=w121:bool, element #8=w122:bool)  [unwired: 8 in]
  n58 = Initialize Array(TRUE, 8 ("dimension size")) -> (w137:bool[])
  n59 = Replace Array Subset(array=w137, new element=w140, index=w141) -> (w139:bool[])
  n60 = Replace Array Subset(array=w137, new element=w123, index=w130) -> (w138:bool[])
  n61 = Replace Array Subset(array=w137, new element=w117, index=w129) -> (w136:bool[])
  n62 = Replace Array Subset(array=w137, new element=w118, index=w128) -> (w135:bool[])
  n63 = Replace Array Subset(array=w137, new element=w119, index=w127) -> (w134:bool[])
  n64 = Replace Array Subset(array=w137, new element=w120, index=w126) -> (w131:bool[])
  n65 = Replace Array Subset(array=w137, new element=w121, index=w125) -> (w132:bool[])
  n66 = Replace Array Subset(array=w137, new element=w122, index=w124) -> (w133:bool[])
  n67 = Compound Arithmetic op=AND(w139, w138, w136, w135, w134, w131, w132, w133) -> (w116:bool[])
  n68 = feedback-in #1(w116) -> ()
  n69 = Select(t=w158, s="gate display until frame complete", f=w116) -> (s? t:f=→"ready for input":bool[])
